vi "Verify Acquisition.vi"(8 "error in (no error)":errorcluster, 11 "CCDCamera in":refnum<class "Sim_CCD.lvclass">) -> (0 "error out":errorcluster, 3 "CCDCamera out":refnum<class "Sim_CCD.lvclass">)   [LabVIEW 2018, in "Sim_CCD.lvclass"]
doc: "Verify if the camera is exposing.\n\nIf the exposure still running, the CCD status will be ACTIVE. Otherwise, it will be IDLE"
uses:
  Sim_CCD.lvclass
  Sim_CCD.lvclass/Sim_CCD.ctl
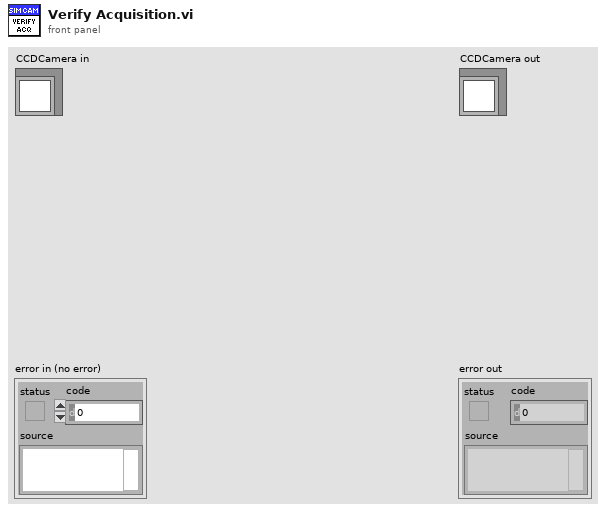
[diagram p1: front panel]
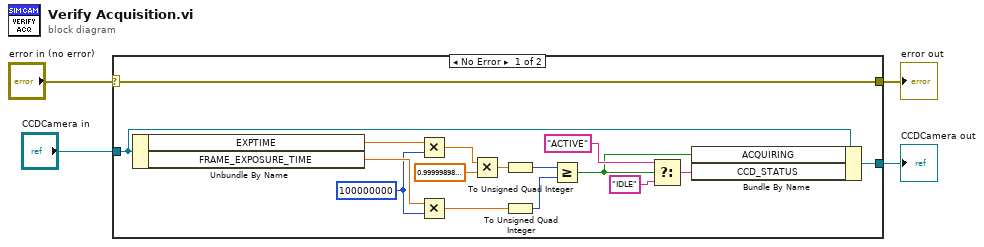
[diagram p0: block diagram]
diagram:
  n1 = case shown="No Error" "error in (no error)" {
    selector: "error in (no error)" -> [w20 w22]
    tunnel: [w20 w22] -> w1
    tunnel: [w15 w21] -> w2
    tunnel: "CCDCamera in" -> [w16 w21]
    frame No Error {
      w11 = 100000000
      n2 = Unbundle By Name(w16) -> ("EXPTIME"=w13:dbl, "FRAME_EXPOSURE_TIME"=w12:sgl)
      n3 = Multiply(x=w13, y=w11) -> (x*y=w7:dbl)
      n4 = Multiply(x=w12, y=w11) -> (x*y=w10:sgl)
      n5 = Multiply(x=w7, y=sgl 0.999999) -> (x*y=w6:dbl)
      n6 = To Unsigned Quad Integer(1:w6) -> (0:w5:u64)
      n7 = To Unsigned Quad Integer(1:w10) -> (0:w9:u64)
      n8 = Greater Or Equal?(x=w5, y=w9) -> (x >= y?=w17:bool)
      n9 = Select(t="ACTIVE", s=w17, f="IDLE") -> (s? t:f=w19:string)
      n10 = Bundle By Name(cluster=w16, "ACQUIRING"=w17, "CCD_STATUS"=w19) -> (w15:refnum<class "Sim_CCD.lvclass">)
    }
    frame Error {
    }
  }
  "error out" <- w1
  "CCDCamera out" <- w2
